vi "Generate Gaussian Kernel.vi"(8 "error in (no error)":errorcluster, 10 "sigma":sgl, 11 "kernel size (odd number)":i32) -> (0 "error out":errorcluster, 3 "Kernel":sgl[][](array[numeric]) format="%.2f")   [LabVIEW 2012]
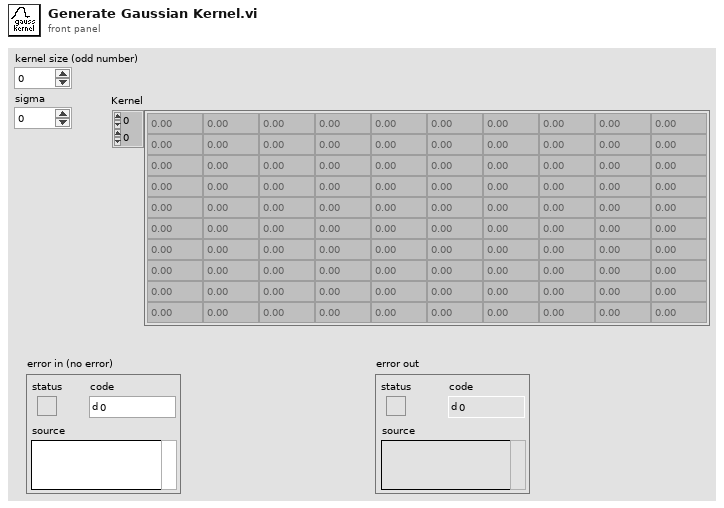
[diagram p1: front panel]
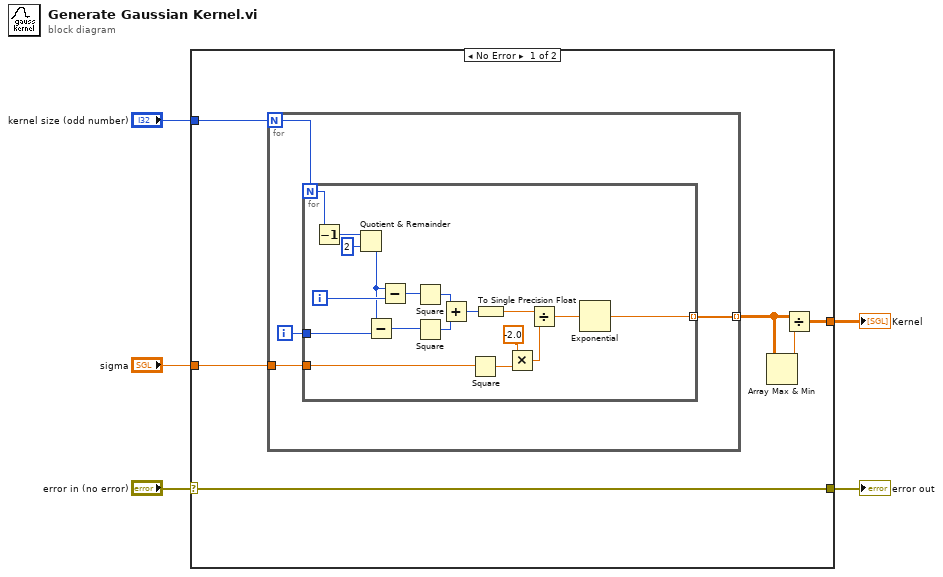
[diagram p0: block diagram]
diagram:
  n1 = case shown="No Error" "error in (no error)" {
    selector: "error in (no error)" -> [w6 w34]
    tunnel: "kernel size (odd number)" -> [w11 _]
    tunnel: "sigma" -> [w10 _]
    tunnel: [w7 _] -> w3
    tunnel: [w6 w34] -> w1
    frame No Error {
      n2 = for {
        N: w11 -> [w15]
        tunnel: w10 -> [w13]
        tunnel: [w12] -> w8 mode=indexing
        i -> [w14]
        n3 = for {
          N: w15 -> [w33]
          tunnel: w14 -> [w28]
          tunnel: w13 -> [w22]
          tunnel: [w16] -> w12 mode=indexing
          i -> [w30]
          n4 = Decrement(x=w33) -> (x-1=w32:i32)
          n5 = Quotient & Remainder(x=w32, y=2) -> (floor(x/y)=w29:i32)  [unwired: 1 out]
          n6 = Subtract(x=w29, y=w28) -> (x-y=w27:i32)
          n7 = Subtract(x=w29, y=w30) -> (x-y=w26:i32)
          n8 = Square(x=w26) -> (x^2=w25:i32)
          n9 = Square(x=w27) -> (x^2=w24:i32)
          n10 = Add(x=w25, y=w24) -> (x+y=w23:i32)
          n11 = Square(x=w22) -> (x^2=w21:sgl)
          n12 = To Single Precision Float(number=w23) -> (single precision float=w19:sgl)
          n13 = Multiply(x=sgl -2.0, y=w21) -> (x*y=w18:sgl)
          n14 = Divide(x=w19, y=w18) -> (x/y=w17:sgl)
          n15 = Exponential(1:w17) -> (0:w16:sgl)
        }
      }
      n16 = Array Max & Min(array=w8) -> (max value=w9:sgl)  [unwired: 3 out]
      n17 = Divide(x=w8, y=w9) -> (x/y=w7:sgl[][])
    }
    frame Error {
    }
  }
  "Kernel" <- w3
  "error out" <- w1
